vi "Initialize Instrument.vi"(8 "error in (no error)":errorcluster, 10 "Reset":bool, 11 "NI USB-6501 in":refnum<class "NI USB-6501.lvclass">) -> (0 "error out":errorcluster, 3 "NI USB-6501 out":refnum<class "NI USB-6501.lvclass">)   [LabVIEW 2020, in "NI USB-6501.lvclass"]
uses:
  NI USB-6501.lvclass
  Controls/Channel.ctl
  <vilib>/DAQmx/write.llb/DAQmx Write (Digital Bool 1Line 1Point).vi
  <vilib>/Utility/config.llb/Read Key (String).vi
  <vilib>/DAQmx/create/channels.llb/DAQmx Create Channel (DO-Digital Output).vi
  <vilib>/DAQmx/miscellaneous.llb/DAQmx Fill In Error Info.vi
  <vilib>/DAQmx/create/channels.llb/DAQmx Create Channel (DI-Digital Input).vi
  <vilib>/Utility/config.llb/NI_LVConfig.lvlib
panel:
  out "configuration file path":path
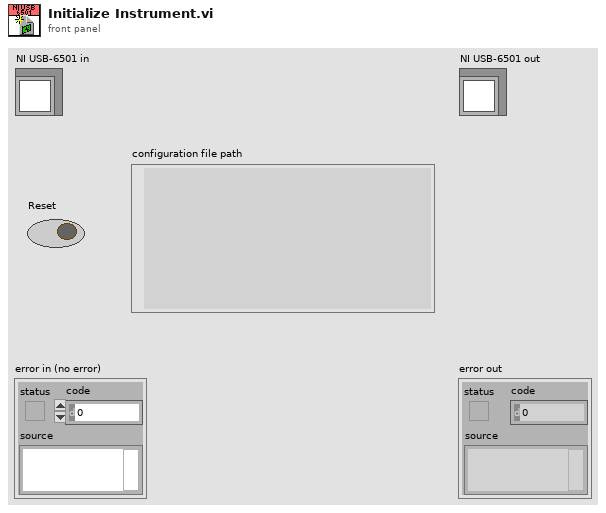
[diagram p1: front panel]
types:
  T1 = typedef "NI USB-6501.lvclass/Channel.ctl" = cluster{"Channel":tag, "Task":refnum<k21>, "Function":string, "Low":string, "High":string, "Direction":enum16{"Input", "Output"}}
  T2 = typedef "NI_LVConfig.lvlib/Config Data RefNum.ctl" = refnum<k1>
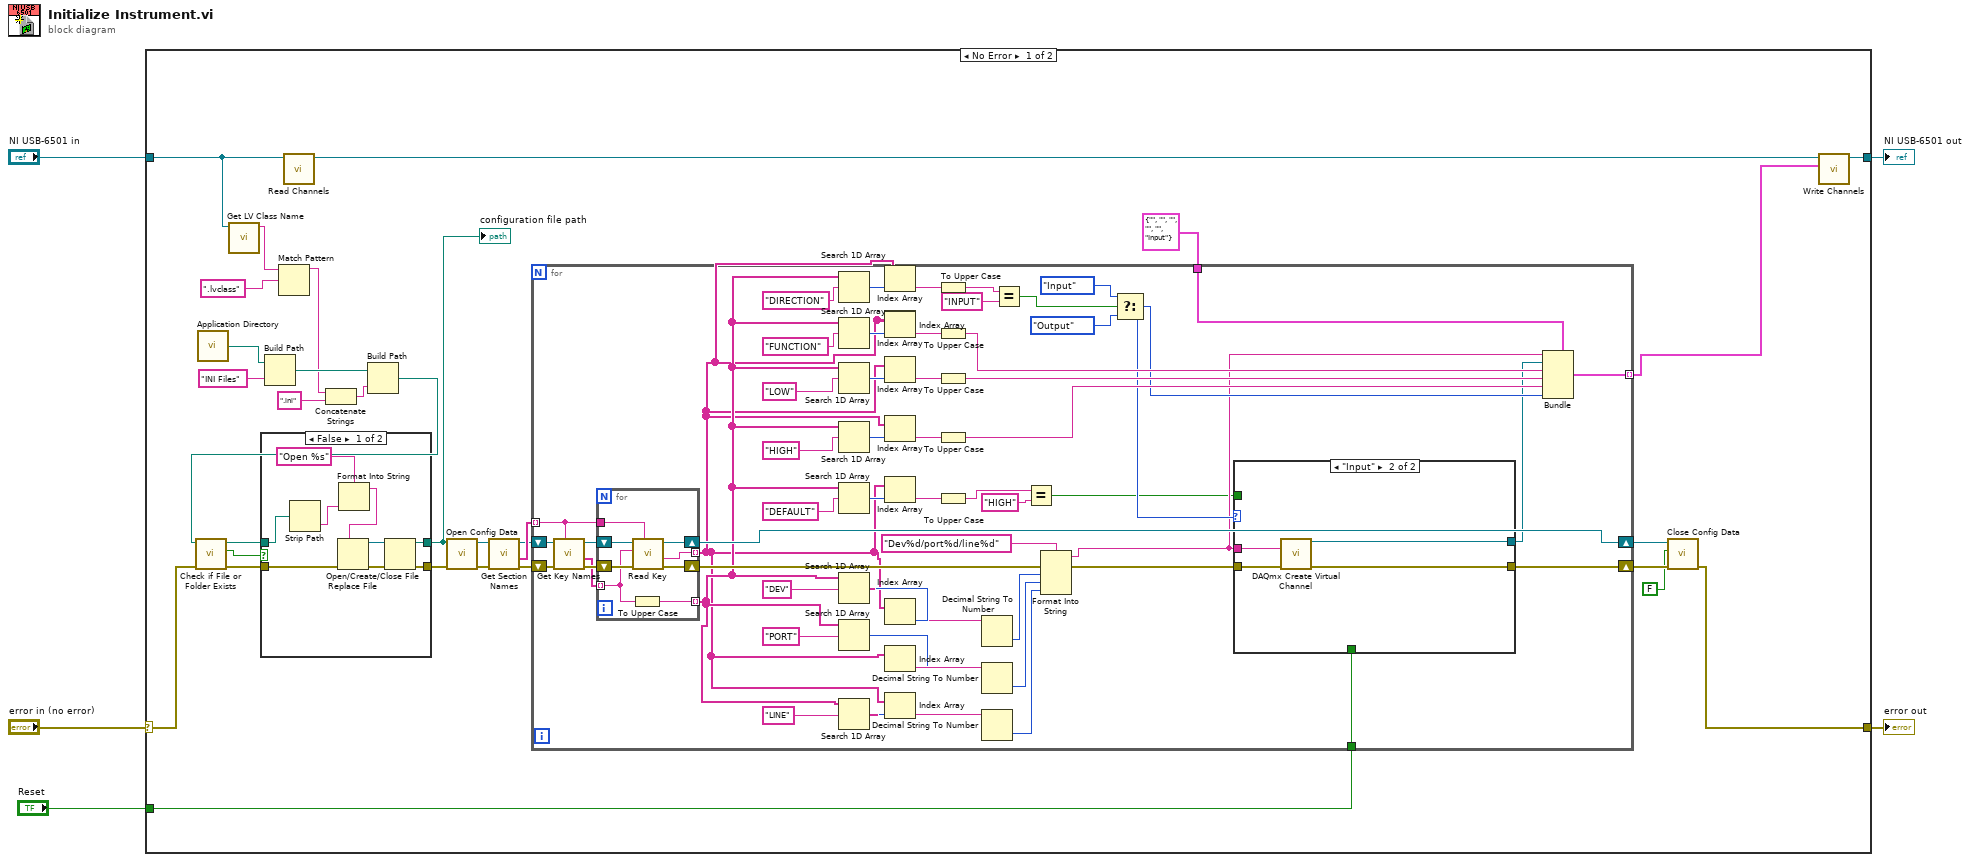
[diagram p0: block diagram]
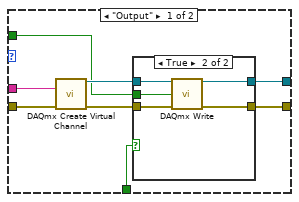
[diagram p3: hidden frame]
diagram:
  n1 = case shown="No Error" "error in (no error)" {
    selector: "error in (no error)" -> [w11 w132]
    tunnel: [w23 w132] -> w4
    tunnel: "NI USB-6501 in" -> [w19 w131]
    tunnel: [w34 w131] -> w2
    tunnel: "Reset" -> [w13 _]
    frame No Error {
      n2 = call <vilib>:"Application Directory.vi"() -> ("Application Directory"=w22:path)
      n3 = call <vilib>:"Get LV Class Name.vi"("object"=w19) -> ("class name"=w18:string)  [unwired: 9 in, 1 out]
      n4 = Build Path(base path=w22, name or relative path="INI Files") -> (appended path=w20:path)
      n5 = Match Pattern(string=w18, regular expression=".lvclass") -> (before substring=w16:string)  [unwired: 1 in, 3 out]
      n6 = call-dynamic "Read Channels.vi"("NI USB-6501 in"=w19) -> ("NI USB-6501 out"=w35:refnum<class "NI USB-6501.lvclass">)  [unwired: 9 in, 1 out]
      n7 = Concatenate Strings(w16, ".ini" ("name or relative path")) -> (w14:string)
      n8 = Build Path(base path=w20, name or relative path=w14) -> (appended path=w12:path)
      n9 = call <vilib>:"Check if File or Folder Exists.vi"("error in (no error)"=w11, "path"=w12) -> ("error out"=w6:errorcluster, "file or folder exists?"=w10:bool, "dup path"=w8:path)  [unwired: 7 in]
      n10 = case shown="False" w10 {
        tunnel: [w41 w46] -> w9
        tunnel: w8 -> [w43 w46]
        tunnel: [w39 w45] -> w7
        tunnel: w6 -> [w44 w45]
        frame False {
          n11 = Strip Path(path=w43) -> (name=w37:string)  [unwired: 1 out]
          n12 = Format Into String(format string="Open %s", w37) -> (resulting string=w36:string)  [unwired: 2 in, 1 out]
          n13 = Open/Create/Replace File(error in=w44, prompt=w36) -> (refnum out=w42:refnum<file>, error out=w40:errorcluster)  [unwired: 4 in, 1 out]
          n14 = Close File(refnum=w42, error in=w40) -> (path=w41:path, error out=w39:errorcluster)
        }
        frame True {
        }
      }
      "configuration file path" <- w9
      n15 = call <vilib>:"Open Config Data.vi"("error in (no error)"=w7, "configuration file path"=w9) -> ("error out"=w28:errorcluster, "refnum"=w27:T2)  [unwired: 7 in, 1 out]
      n16 = call <vilib>:"Get Section Names.vi"("error in (no error)"=w28, "refnum"=w27) -> ("error out"=w30:errorcluster, "section names"=w33:string[], "refnum out"=w29:T2)  [unwired: 7 in]
      n17 = for {
        tunnel: w33 -> [w97] mode=indexing
        shift-right: [w99] -> w31
        shift-left: w29 -> [w103]
        shift-right: [w52] -> w32
        shift-left: w30 -> [w102]
        tunnel: T1 {"Channel"="", "Task"="", "Function"="", "Low"="", "High"="", "Direction"=enum."Input"} ("Channel") -> [w77]
        tunnel: [w64] -> w24 mode=indexing
        tunnel: w13 -> [w47]
        n18 = call <vilib>:"Get Key Names.vi"("section"=w97, "error in (no error)"=w102, "refnum"=w103) -> ("error out"=w100:errorcluster, "key names"=w98:string[], "refnum out"=w101:T2)  [unwired: 5 in, 1 out]
        n19 = for {
          tunnel: w98 -> [w124] mode=indexing
          tunnel: w97 -> [w125]
          shift-right: [w128] -> w99
          shift-left: w101 -> [w130]
          shift-right: [w127] -> w83
          shift-left: w100 -> [w129]
          tunnel: [w126] -> w54 mode=indexing
          tunnel: [w123] -> w60 mode=indexing
          n20 = To Upper Case(1:w124) -> (0:w123:string)
          n21 = call-poly <vilib>:"Read Key.vi"("section"=w125, "error in (no error)"=w129, "key"=w124, "refnum"=w130) -> ("error out"=w127:errorcluster, "value"=w126:string, "refnum out"=w128:T2)  [unwired: 4 in, 1 out]
        }
        n22 = Search 1D Array(1D array=w60, element="DIRECTION") -> (index of element=w61:i32)  [unwired: 1 in]
        n23 = Search 1D Array(1D array=w60, element="FUNCTION") -> (index of element=w72:i32)  [unwired: 1 in]
        n24 = Search 1D Array(1D array=w60, element="LOW") -> (index of element=w75:i32)  [unwired: 1 in]
        n25 = Search 1D Array(1D array=w60, element="HIGH") -> (index of element=w74:i32)  [unwired: 1 in]
        n26 = Search 1D Array(1D array=w60, element="DEFAULT") -> (index of element=w82:i32)  [unwired: 1 in]
        n27 = Search 1D Array(1D array=w60, element="DEV") -> (index of element=w94:i32)  [unwired: 1 in]
        n28 = Search 1D Array(1D array=w60, element="PORT") -> (index of element=w90:i32)  [unwired: 1 in]
        n29 = Search 1D Array(1D array=w60, element="LINE") -> (index of element=w87:i32)  [unwired: 1 in]
        n30 = Index Array(array=w54, index=w61) -> (element=w62:string)
        n31 = Index Array(array=w54) -> ()  [unwired: 1 in, 1 out]
        n32 = Index Array(array=w54, index=w72) -> (element=w71:string)
        n33 = Index Array(array=w54, index=w75) -> (element=w76:string)
        n34 = Index Array(array=w54, index=w74) -> (element=w73:string)
        n35 = Index Array(array=w54, index=w82) -> (element=w79:string)
        n36 = Index Array(array=w54, index=w94) -> (element=w93:string)
        n37 = Index Array(array=w54, index=w90) -> (element=w91:string)
        n38 = Index Array(array=w54, index=w87) -> (element=w86:string)
        n39 = To Upper Case(1:w62) -> (0:w59:string)
        n40 = To Upper Case(1:w71) -> (0:w65:string)
        n41 = To Upper Case(1:w76) -> (0:w66:string)
        n42 = To Upper Case(1:w73) -> (0:w67:string)
        n43 = To Upper Case(1:w79) -> (0:w78:string)
        n44 = Decimal String To Number(string=w93) -> (number=w92:i32)  [unwired: 2 in, 1 out]
        n45 = Decimal String To Number(string=w91) -> (number=w85:i32)  [unwired: 2 in, 1 out]
        n46 = Decimal String To Number(string=w86) -> (number=w84:i32)  [unwired: 2 in, 1 out]
        n47 = Equal?(x=w59, y="INPUT") -> (x = y?=w55:bool)
        n48 = Equal?(x=w78, y="HIGH") -> (x = y?=w48:bool)
        n49 = Format Into String(format string="Dev%d/port%d/line%d", error in=w83, w92, w85, w84) -> (resulting string=w50:string, error out=w53:errorcluster)  [unwired: 1 in]
        n50 = Select(t=enum16{"Input", "Output"}."Input" ("Direction"), s=w55, f=enum16{"Input", "Output"}."Output" ("Direction")) -> (s? t:f=w51:enum16{"Input", "Output"})
        n51 = case shown="\"Input\"" w51 {
          tunnel: w50 -> [w111 w119]
          tunnel: [w106 w122] -> w49
          tunnel: [w107 w121] -> w52
          tunnel: w53 -> [w110 w120]
          tunnel: w48 -> [w105 _]
          tunnel: w47 -> [w104 _]
          frame "Output" {
            n52 = call-poly <vilib>:"DAQmx Create Virtual Channel.vi"("lines"=w111, "error in"=w110) -> ("task out"=w109:refnum<k21>, "error out"=w108:errorcluster)  [unwired: 12 in]
            n53 = case shown="True" w104 {
              tunnel: w109 -> [w112 w118]
              tunnel: w108 -> [w113 w117]
              tunnel: [w113 w116] -> w107
              tunnel: [w112 w115] -> w106
              tunnel: w105 -> [_ w114]
              frame False {
              }
              frame True {
                n54 = call-poly <vilib>:"DAQmx Write.vi"("task/channels in"=w118, "data"=w114, "error in"=w117) -> ("task out"=w115:refnum<k21>, "error out"=w116:errorcluster)  [unwired: 10 in, 1 out]
              }
            }
          }
          frame "Input" {
            n55 = call-poly <vilib>:"DAQmx Create Virtual Channel.vi"("lines"=w119, "error in"=w120) -> ("task out"=w122:refnum<k21>, "error out"=w121:errorcluster)  [unwired: 12 in]
          }
        }
        n56 = Bundle(cluster=w77, "Channel"=w50, "Task"=w49, "Function"=w65, "Low"=w66, "High"=w67, "Direction"=w51) -> (w64:T1)
      }
      n57 = call <vilib>:"Close Config Data.vi"("error in (no error)"=w32, "write file if changed (T)"=FALSE, "refnum"=w31) -> ("error out"=w23:errorcluster)  [unwired: 7 in, 1 out]
      n58 = call-dynamic "Write Channels.vi"("Channels"=w24, "NI USB-6501 in"=w35) -> ("NI USB-6501 out"=w34:refnum<class "NI USB-6501.lvclass">)  [unwired: 9 in]
    }
    frame Error {
    }
  }
  "error out" <- w4
  "NI USB-6501 out" <- w2
